vi "Send Report Iterations End.vi"(7 "Priority":T2=enum."Normal" caption="Message Priority (Normal)", 8 "error in (no error)":errorcluster, 9 "Stop Reason":T1, 10 "Caller Error Handler":refnum<class "Iterator Report Iterations End Msg.lvclass">, 11 "Caller Enqueuer in":refnum<class "Message Enqueuer.lvclass">) -> (0 "error out":errorcluster, 3 "Caller Enqueuer out":refnum<class "Message Enqueuer.lvclass">)   [LabVIEW 2021, in "Iterator Actor.lvlib" / "Iterator Report Iterations End Msg.lvclass"]
doc: "Sends the <b>Iterator Actor 2.lvlib:Stop Iterate Msg.lvclass</b> message.\n\nThis message will call <b>Stop Iterate.vi</b> on the <b>Iterator Actor 2.lvlib:Iterator Actor 2.lvclass</b> actor.\n\n<b>Stop Iterate.vi Description</b>"
uses:
  Iterator Report Iterations End Msg.lvclass
  <vilib>/ActorFramework/Message Enqueuer/Message Enqueuer.lvclass
  <vilib>/ActorFramework/Message Enqueuer/Message Priority.ctl
  C:/Program Files/National Instruments/LabVIEW 2021/vi.lib/ActorFramework/Message/Message.lvclass
  Iterator Report Iterations End Msg.lvclass/Iterator Report Iterations End Msg.ctl
  <vilib>/ActorFramework/Message Enqueuer/Message Enqueuer.lvclass/Message Enqueuer.ctl
  <vilib>/ActorFramework/Message Priority Queue/Priority Enqueue.vi
  Abstract Iterator Actor/Stop Reason.ctl
  Abstract Iterator Actor/Abstract Iterator Actor.lvclass
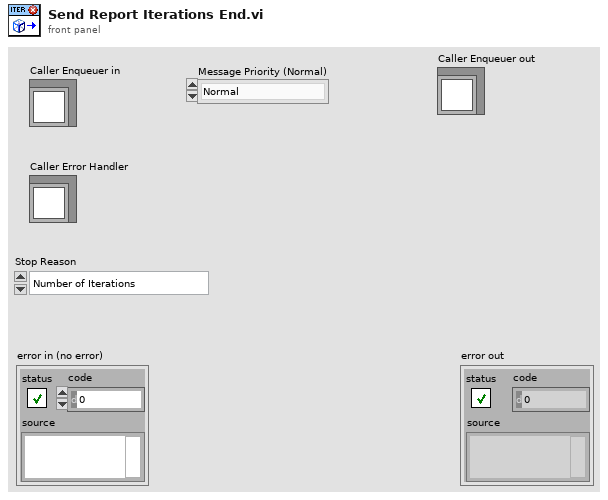
[diagram p1: front panel]
types:
  T1 = typedef "Iterator Actor.lvlib/Abstract Iterator Actor.lvclass/Stop Reason.ctl" = enum16{"Number of Iterations", "Time Elapsed", "Stopped Internally", "Stopped Externally"}
  T2 = typedef "Actor Framework.lvlib/Message Enqueuer.lvclass/Message Priority.ctl" = enum16{"Low", "Normal", "High"}
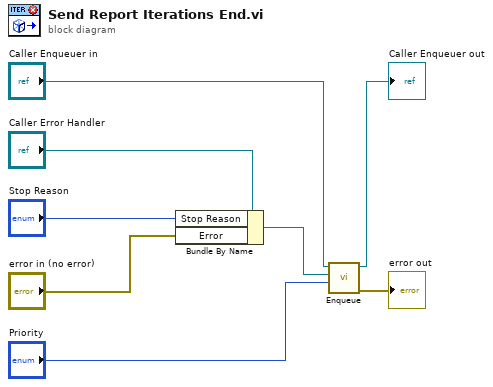
[diagram p0: block diagram]
diagram:
  n1 = Bundle By Name(cluster="Caller Error Handler", "Stop Reason"="Stop Reason", "Error"="error in (no error)") -> (w3:refnum<class "Iterator Report Iterations End Msg.lvclass">)
  n2 = call <vilib>:"Enqueue.vi"("Message Priority (Normal)"="Priority", "Message"=w3, "Message Enqueuer in"="Caller Enqueuer in") -> ("error out"=→"error out":errorcluster, "Message Enqueuer out"=→"Caller Enqueuer out":refnum<class "Message Enqueuer.lvclass">)  [unwired: 7 in]
